vi "loop stop global.vi"() -> ()   [LabVIEW 2022 SP3]
panel:
  in  "Loop Stop":bool
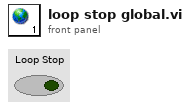
[diagram p1: front panel]
diagram:
